vi "Main.vi"() -> ()   [LabVIEW 2013] (continued)
            n2550 = property on="Material Save" class="Bool"("DisabledEnum"=w4223) -> ()  [unwired: 2 in, 2 out]
            n2551 = property class="Clust (strict)"(reference=w4231, "Value"=w4228) -> (reference out=w4227:refnum<vi>)  [unwired: 1 in, 1 out]
            n2552 = local read "DB - Master Data Load"() -> (w4236:bool)
            n2553 = case shown="True" w4236 {
              tunnel: w4227 -> [_ w4239]
              tunnel: w4225 -> [_ w4241]
              frame False {
              }
              frame True {
                w4240 = FALSE  # Include Inactive
                # "Updates Picture"
                # "We will update the [ShortDescription] later during Revision Toggle.\nActually no problem updating here also, but easier to debug code if we\nupdate only in one location."
                # "Updates Rev ComboBox"
                # "Use DB"
                n2554 = local read "Logon"() -> (w4244:T21)
                n2555 = Unbundle By Name(w4244) -> ("LanguageID"=w4243:string)
                n2556 = call "DB - [MasterData].[Material].vi"("DB - Master Data Material Enum"=DB_-_Master_Data_Material_Enum."SELECT [ShortDescription]", "Include Inactive"=w4240, "SRTRS.MasterData.SAPMaterial/Material"="SRTRS.MasterData.SAPMaterial", "[LanguageId]"=w4243, "Update [ShortDescription] to Cluster"=FALSE, "Clust Refnum"=w4239) -> ("SUMMARY"=w4238:errorcluster)  [unwired: 5 in, 4 out]
                n2557 = local write "DB"(w4238) -> ()
                n2558 = disable-structure shown="Disabled" {
                  disable-tunnel: w4241 -> [w4251 _]
                  disable-tunnel: w4238 -> [w4248 _]
                  frame Disabled {
                    n2559 = control-ref of="Master Data Rev"() -> (w4250:refnum<vi>)
                    n2560 = property class="CmbBox"(reference=w4250, error in=w4248, "Value"="") -> (error out=w4247:errorcluster)  [unwired: 1 out]
                    n2561 = property on="Revision Toggle" class="Str"(error in=w4247, "Val(Sgnl)"=w4251) -> (error out=w4249:errorcluster)  [unwired: 1 in, 1 out]
                    n2562 = local write "Property Node Error"(w4249) -> ()
                  }
                  frame Enabled {
                  }
                }
              }
            }
          }
          frame True {
            # "Blank"
          }
        }
      }
      event "Material.Inactive": Value Change {
        n2563 = event-data() -> ("NewVal"=w4252:bool)  [unwired: 1 in, 5 out]
        n2564 = case shown="True" w4252 {
          frame False {
          }
          frame True {
            n2565 = property on="Master Data Material" class="CmbBox"() -> ("Value"=w4257:string)  [unwired: 2 in, 2 out]
            n2566 = property on="Master Data Rev" class="CmbBox"() -> ("Value"=w4256:string)  [unwired: 2 in, 2 out]
            n2567 = call "String - Create comma seperated String.vi"("B"=w4256, "A"=w4257) -> ("A, B , C (auto comma)"=w4255:string)  [unwired: 9 in]
            n2568 = call "Msgbox - Message Handler.vi"("Short Description (When DB Not Available)"="Inactive Material", "Description (When DB Not Available)"=" cannot be used after inactive. Do you wish to proceed?", "Pre-Description"=w4255, "<.?....> Message Code"="<W 504>") -> ("MHandler Error"=w4253:errorcluster, "OK Out"=w4254:bool)  [unwired: 5 in, 1 out]
            n2569 = local write "MHandler"(w4253) -> ()
            n2570 = property on="Inactive" class="Bool (strict)"("Value"=w4254) -> ()  [unwired: 2 in, 2 out]
          }
        }
      }
      event "Revision Toggle": Value Change {
        # "Called by who?\nIf called by Rev"
        # "Called by either \nItem Details.Order No OR\nItem Details.Revision OR\nMaterial.Master Data Rev"
        n2571 = event-data() -> ("NewVal"=w4261:string)  [unwired: 1 in, 5 out]
        n2572 = case shown="\"Master Data Material\", \"Master Data Rev\"" w4261 {
          tunnel: [w4332 w4345] -> w4271
          tunnel: [w4339 w4344] -> w4269
          tunnel: [w4338 w4343] -> w4270
          tunnel: [w4330 w4342] -> w4267
          tunnel: [w4329 w4341] -> w4266
          tunnel: [w4328 w4340] -> w4262
          frame "Material", "Order No", "Revision", Default {
            w4329 = FALSE  # Include Inactive
            # "Use Buffer because Revsion in Part Details's Item Details  is \n different from Cluster of Rev in Material"
            # "Order No & Parts Details.Revision\nFrom Parts Detail"
            n2573 = control-ref of="Material"() -> (w4333:refnum<vi>)
            n2574 = control-ref of="Setup Thermocouple Location"() -> (w4338:refnum<vi>)
            n2575 = control-ref of="Material Description"() -> (w4339:refnum<vi>)
            n2576 = control-ref of="Material Buffer"() -> (w4334:refnum<vi>)
            n2577 = property on="Revision" class="CmbBox"() -> ("Value"=w4328:string)  [unwired: 2 in, 2 out]
            n2578 = property class="Clust (strict)"(reference=w4334) -> (reference out=w4337:refnum<vi>, "Value"=w4335:T12)  [unwired: 1 in, 1 out]
            n2579 = property on="Material" class="CmbBox"(reference=w4333) -> (reference out=w4332:refnum<vi>, "Value"=w4331:string)  [unwired: 1 in, 1 out]
            n2580 = Bundle By Name(cluster=w4335, "Master Data Material"=w4331, "Master Data Rev"=w4328) -> (w4336:T12)
            n2581 = property class="Clust (strict)"(reference=w4337, "Value"=w4336) -> (reference out=w4330:refnum<vi>)  [unwired: 1 in, 1 out]
          }
          frame "Master Data Material", "Master Data Rev" {
            w4341 = TRUE  # Include Inactive
            # "From Material.Master Data Rev"
            n2582 = control-ref of="Master Data Material Description"() -> (w4344:refnum<vi>)
            n2583 = control-ref of="Master Data Thermocouple Location"() -> (w4343:refnum<vi>)
            n2584 = control-ref of="Master Data Material"() -> (w4345:refnum<vi>)
            n2585 = control-ref of="Material"() -> (w4342:refnum<vi>)
            n2586 = property on="Master Data Rev" class="CmbBox"() -> ("Value"=w4340:string)  [unwired: 2 in, 2 out]
          }
        }
        n2587 = local read "DB - Master Data Load"() -> (w4268:bool)
        n2588 = property on="Material" class="CmbBox"(reference=w4271) -> ("Value"=w4272:string)  [unwired: 1 in, 2 out]
        n2589 = case shown="True" w4268 {
          tunnel: [w4279 w4314] -> w4273
          tunnel: w4272 -> [w4281 _]
          tunnel: w4269 -> [w4280 w4301]
          tunnel: w4267 -> [_ w4313]
          tunnel: w4266 -> [_ w4312]
          tunnel: [w4277 w4311] -> w4265
          tunnel: [w4275 w4310] -> w4264
          tunnel: w4262 -> [w4274 _]
          frame False {
            w4293 = "_" ("string")
            n2590 = Concatenate Strings(w4281, w4293, w4274, w4293) -> (w4286:string)
            n2591 = local read "MasterData\\JPG"() -> (w4290:path)
            n2592 = Concatenate Strings(w4286, "*.jpg" ("string")) -> (w4285:string)
            n2593 = List Folder(path=w4290, pattern=w4285) -> (filenames=w4292:string[])  [unwired: 2 in, 3 out]
            n2594 = Index Array(array=w4292, index=0) -> (element=w4288:string)
            n2595 = Build Path(base path=w4290, name or relative path=w4288) -> (appended path=w4289:path)
            n2596 = Match Pattern(string=w4288, regular expression=w4286) -> (after substring=w4284:string)  [unwired: 1 in, 3 out]
            n2597 = Match Pattern(string=w4284, regular expression="[.]") -> (before substring=w4282:string)  [unwired: 1 in, 3 out]
            n2598 = property class="Str"(reference=w4280, "Value"=w4282) -> (reference out=w4278:refnum<vi>)  [unwired: 1 in, 1 out]
            n2599 = call <vilib>:"Check if File or Folder Exists.vi"("path"=w4289) -> ("file or folder exists?"=w4279:bool, "dup path"=w4276:path)  [unwired: 8 in, 1 out]
            n2600 = case shown="True" w4279 {
              tunnel: w4278 -> [w4294 _]
              tunnel: w4276 -> [_ w4297]
              tunnel: [_ w4296] -> w4277
              frame False {
                # "File Does Not Exist"
                n2601 = invoke class="Str" method="Reinit To Default"(reference=w4294) -> ()  [unwired: 2 in, 3 out]
              }
              frame True {
                n2602 = local write "MasterData Image File Path"(w4297) -> ()
                n2603 = call <vilib>:"Read JPEG File.vi"("path to JPEG file"=w4297) -> ("error out"=→"Material Image File":errorcluster, "image data"=w4296:T40)  [unwired: 8 in, 1 out]
              }
            }
            n2604 = Path To String(path=w4276) -> (string=w4275:string)
          }
          frame True {
            # "Update Description only if Rev is Blank"
            # "Use DB"
            n2605 = local read "Logon"() -> (w4308:T21)
            n2606 = Unbundle By Name(w4308) -> ("LanguageID"=w4307:string)
            n2607 = call "DB - [MasterData].[Material].vi"("DB - Master Data Material Enum"=DB_-_Master_Data_Material_Enum."SELECT [Description], [ImageFile]", "Include Inactive"=w4312, "[LanguageId]"=w4307, "Clust Refnum"=w4313) -> ("image data"=w4311:T40, "ImageFile OK"=w4314:bool, "Material File"=w4309:path, "SUMMARY"=w4316:errorcluster)  [unwired: 7 in, 1 out]
            n2608 = property class="Clust (strict)"(reference=w4313, error in=w4316) -> (error out=w4304:errorcluster, "Value"=w4315:T12)  [unwired: 1 out]
            n2609 = Unbundle By Name(w4315) -> ("Master Data Material Description"=w4302:string)
            n2610 = disable-structure shown="Enabled" {
              disable-tunnel: w4302 -> [w4325 _]
              disable-tunnel: [w4324 T30."Enabled" ("Disabled")] -> w4299
              disable-tunnel: [w4318 u32 16777215] -> w4298
              frame Disabled {
                n2611 = Empty String/Path?(string/path=w4325) -> (empty?=w4321:bool)
                n2612 = Select(t=u32 16777215, s=w4321, f=u32 16250871) -> (s? t:f=w4318:u32)
                n2613 = Select(t=T30."Enabled" ("Disabled"), s=w4321, f=T30."Disabled" ("Disabled")) -> (s? t:f=w4324:T30)
              }
              frame Enabled {
              }
            }
            n2614 = local write "MasterData Image File Path"(w4309) -> ()
            n2615 = local read "Logon Extra"() -> (w4306:T25)
            n2616 = property class="Str"(reference=w4301, "DisabledEnum"=w4299, "Text.BGColor"=w4298) -> (reference out=w4300:refnum<vi>)  [unwired: 1 in, 1 out]
            n2617 = Unbundle By Name(w4306) -> ("IsUnicode"=w4305:bool)
            n2618 = call "Tool_Unicode Update String.vi"("Interpret as Unicode (T)"=w4305, "error in (no error)"=w4304, "String Value"=w4302, "String Control Reference"=w4300) -> ("error out"=w4303:errorcluster)  [unwired: 4 in, 1 out]
            n2619 = local write "Material Image File"(w4303) -> ()
            n2620 = Path To String(path=w4309) -> (string=w4310:string)
          }
        }
        n2621 = case shown="True" w4273 {
          tunnel: w4270 -> [w4348 w4355]
          tunnel: w4265 -> [_ w4352]
          tunnel: w4264 -> [_ w4351]
          tunnel: [w4346 w4350] -> w4263
          frame False {
            # "No Image"
            n2622 = disable-structure shown="Disabled" {
              frame Disabled {
                n2623 = property on="Material Save" class="Bool"("DisabledEnum"=T30."Disabled and Grayed Out" ("Disabled")) -> ()  [unwired: 2 in, 2 out]
              }
              frame Enabled {
              }
            }
            n2624 = invoke class="Pict" method="Reinit To Default"(reference=w4348) -> (error out=w4346:errorcluster)  [unwired: 2 in, 2 out]
            n2625 = property on="Material Copy" class="Bool"("DisabledEnum"=T30."Disabled and Grayed Out" ("Disabled")) -> ()  [unwired: 2 in, 2 out]
          }
          frame True {
            # "Valid Image File"
            n2626 = disable-structure shown="Disabled" {
              frame Disabled {
                n2627 = property on="Material Save" class="Bool"("DisabledEnum"=T30."Enabled" ("Disabled")) -> ()  [unwired: 2 in, 2 out]
              }
              frame Enabled {
              }
            }
            n2628 = call <vilib>:"Draw Flattened Pixmap.vi"("image data"=w4352, "picture"=picture data[5B]) -> ("new picture"=w4356:picture)  [unwired: 7 in]
            n2629 = property on="Material Copy" class="Bool"("DisabledEnum"=T30."Enabled" ("Disabled")) -> ()  [unwired: 2 in, 2 out]
            n2630 = property on="Property Node" class="Pict"(reference=w4355, "Value"=w4356, "Desc"=w4351) -> (error out=w4350:errorcluster)  [unwired: 1 in, 1 out]
          }
        }
        n2631 = local write "Material Image File"(w4263) -> ()
      }
    }
    "UI Event" <- w479
  }
  n2632 = while {
    shift-right: [w4366] -> _
    shift-left: w25 -> [w4363]
    shift-right: [w4367] -> w7
    shift-left: w24 -> [w4372]
    shift-right: [w4368] -> _
    shift-left: w15 -> [w4369]
    tunnel: w20 -> [_]
    shift-left: w1 -> [w4364]
    shift-right: [w4361] -> _
    shift-left: w13 -> [w4362]
    shift-right: [w4360] -> _
    shift-left: w12 -> [w4359]
    stop <- w4365 stop-if-true
    # "StateMachine For MainProcess                                                         StateMachine For MainProcess                                                         StateMachine For MainProcess                                                         StateMachine For MainProcess                                                         StateMachine For MainProcess                                                         StateMachine For MainProcess                                                         StateMachine For MainProcess"
    n2633 = case shown="\"END Recipe\"" w4363 {
      selector: w4363 -> [w4391 _ _ _ w5684 _ _ _ _ w6675]
      tunnel: [w4382 w5238 Enum_-_SRTRS_State."BEGIN Process" ("Enum") Enum_-_SRTRS_State."RUNNING Process" ("Enum") w5685 Enum_-_SRTRS_State."Spare Enum" ("Enum") Enum_-_SRTRS_State."END Recipe" ("Enum") Enum_-_SRTRS_State."READY TO START" ("Enum") w6608 w6675] -> w4371
      tunnel: [w4388 w5228 _ w5569 w5670 w6212 _ w6264 _ _] -> w4367
      tunnel: w4372 -> [_ _ _ _ _ w6212 _ _ w6606 _]
      tunnel: [_ _ _ _ _ _ _ _ w6607 TRUE] -> w4365
      tunnel: w4369 -> [w4385 _ _ _ w5661 _ _ _ w6604 _]
      tunnel: [w4389 0 _ w5565 w5678 _ 0 _ w6604 _] -> w4368
      tunnel: w4364 -> [w4390 _ _ _ _ _ _ _ w6605 _]
      tunnel: w4362 -> [_ _ _ _ w5676 _ _ _ w6603 _]
      tunnel: [_ _ _ ET3500_Program_Status."Wait For RUN" w5675 _ _ _ w6603 _] -> w4361
      tunnel: [_ _ _ _ w5673 _ _ _ w6602 _] -> w4360
      tunnel: w4359 -> [_ _ _ _ w5672 _ _ _ w6602 _]
      frame "READY TO START", Default {
        (unwired) FALSE  # RecoveryFlag only checked at "Execute" Page
        # "This wil be checked again at \"Start Cycle\" to prevent resending of DAQ Start"
        # "Setup, Default\nLogon\nExecute"
        n2634 = flat-sequence {
          frame #0 {
            # "Check if Transaction Number is Empty"
            n2635 = local read "Transaction No"() -> (w4397:string)
            n2636 = Empty String/Path?(string/path=w4397) -> (empty?=w4396:bool)
            n2637 = Select(t=T30."Disabled and Grayed Out" ("Disabled"), s=w4396, f=T30."Enabled" ("Disabled")) -> (s? t:f=w4398:T30)
            n2638 = property on="Recipe Start" class="Bool"("DisabledEnum"=w4398) -> ()  [unwired: 2 in, 2 out]
            n2639 = property on="Close" class="Bool (strict)"("DisabledEnum"=T30."Enabled" ("Disabled")) -> ()  [unwired: 2 in, 2 out]
          }
        }
        n2640 = local read "Tab Body"() -> (w4387:T1)
        n2641 = Equal?(x=w4391, y=w4390) -> (x = y?=w4386:bool)
        n2642 = case shown="\"Logon\"" w4387 {
          selector: w4387 -> [_ w4981]
          tunnel: [w4406 w4986] -> w4389
          tunnel: [w4405 w4985] -> w4383
          tunnel: [_ w4984] -> w4388
          tunnel: w4386 -> [_ _]
          tunnel: w4385 -> [_ _]
          frame "Logon" {
            w4405 = FALSE  # RecoveryFlag only checked at "Setup" Tab
            w4406 = 0  # Resets Sample/ch count
            # "\"ini\" Settings to be loaded here"
            n2643 = local read "Logon OK"() -> (w4404:bool)
            n2644 = case shown="True" w4404 {
              frame False {
                # "Check Logon OK"
                n2645 = flat-sequence {
                  tunnel: [w4413] -> w4409
                  tunnel: w4409 -> [w4420]
                  tunnel: [w4421] -> w4408
                  tunnel: [w4420] -> w4407
                  tunnel: w4408 -> [w4422]
                  tunnel: w4407 -> [w4423]
                  frame #0 {
                    n2646 = control-ref of="Logon OK"() -> (w4411:refnum<vi>)
                    n2647 = control-ref of="[RawDataReport]"() -> (w4410:refnum<vi>)
                    n2648 = control-ref of="Logon"() -> (w4412:refnum<vi>)
                    n2649 = control-ref of="Logon Extra"() -> (w4416:refnum<vi>)
                    n2650 = control-ref of="[TabUserAccess]"() -> (w4414:refnum<vi>)
                    n2651 = local read "Logon UI"() -> (w4413:refnum<vi>)
                    n2652 = Build Array(w4411, w4412, w4416, w4414, w4410) -> (w4415:refnum<vi>[])
                    n2653 = for {
                      tunnel: w4413 -> [w4419]
                      tunnel: w4415 -> [w4418] mode=indexing
                      n2654 = call "subPanel - Read Value.vi"("subPanel Ref"=w4419, "CtlRef"=w4418) -> ("Error Out"=w4417:errorcluster)  [unwired: 6 in, 3 out]
                      n2655 = local write "SubPanel"(w4417) -> ()
                    }
                  }
                  frame #1 {
                    # "SET GLOBAL SRTRS to Logon Parameters"
                    n2656 = local read "Logon OK"() -> (w4421:bool)
                  }
                  frame #2 {
                    n2657 = case shown="True" w4422 {
                      tunnel: w4423 -> [_ w4431]
                      frame False {
                      }
                      frame True {
                        # "Logon UI should already be closed"
                        n2658 = control-ref of="Logon UI"() -> (w4432:refnum<vi>)
                        n2659 = Close Reference(reference=w4431) -> (error out=w4433:errorcluster)  [unwired: 1 in]
                        n2660 = invoke on="Invoke Node" class="SubPnl" method="Remove VI"(reference=w4432, error in=w4433) -> (error out=→"SubPanel":errorcluster)  [unwired: 1 in, 2 out]
                        n2661 = global write "Global SRTRS.vi" "[RawDataReport]"("[RawDataReport]") -> ()
                        n2662 = global write "Global SRTRS.vi" "Logon Extra"("Logon Extra") -> ()
                        n2663 = global write "Global SRTRS.vi" "Logon"("Logon") -> ()
                        n2664 = Unbundle By Name("Logon") -> ("PlantID"=w4428:string, "UserID"=w4426:string)
                        n2665 = disable-structure shown="Enabled" {
                          disable-tunnel: w4426 -> [w4436 _]
                          disable-tunnel: "Logon Extra" -> [_ _]
                          disable-tunnel: "Logon" -> [_ _]
                          frame Enabled {
                            n2666 = call "Msgbox - Message Handler.vi"("Short Description (When DB Not Available)"="Logon Successful", "Description (When DB Not Available)"=" logon successful." ("Short Description (When DB Not Available)"), "Pre-Description"=w4436, "<.?....> Message Code"="<I 101>") -> ("MHandler Error"=w4437:errorcluster)  [unwired: 5 in, 2 out]
                            n2667 = local write "MHandler"(w4437) -> ()
                          }
                          frame Disabled {
                          }
                        }
                        n2668 = local write "User"(w4426) -> ()
                        n2669 = String Length(string=w4428) -> (length=w4427:i32)
                        n2670 = case shown="0" w4427 {
                          tunnel: "Logon Extra" -> [_ _]
                          frame 0 {
                            w4439 = FALSE
                            # "No PlantId\nDB Failed. Disable all DB."
                            n2671 = local write "DB - Master Data Save"(w4439) -> ()
                            n2672 = local write "DB - Master Data Load"(w4439) -> ()
                            n2673 = local write "DB - Setup Item (Part Details)"(w4439) -> ()
                            n2674 = local write "DB - Transaction"(w4439) -> ()
                            n2675 = local write "DB - Logon"(w4439) -> ()
                            n2676 = local write "DB - Report"(w4439) -> ()
                            n2677 = local write "DB - Message"(w4439) -> ()
                            n2678 = local write "DB - Active Process"(w4439) -> ()
                            n2679 = global write "Global SRTRS.vi" "DB Available"(w4439) -> ()
                            n2680 = call "Msgbox - Message Handler.vi"("Short Description (When DB Not Available)"="Database Not Available", "Description (When DB Not Available)"="Switching to standalone mode" ("Short Description (When DB Not Available)"), "<.?....> Message Code"="<E 107>") -> ("MHandler Error"=w4444:errorcluster, "OK Out"=w4442:bool)  [unwired: 6 in, 1 out]
                            n2681 = local write "MHandler"(w4444) -> ()
                            n2682 = case shown="True" w4442 {
                              frame False {
                                # "Cancel"
                                n2683 = local write "Tab Body"(Enum_-_Tabs."Logon" ("Tab Body")) -> ()
                                n2684 = local write "Logon OK"(FALSE ("Logon OK")) -> ()
                                n2685 = property on="Close" class="Bool (strict)"("BoolText.Text"="Close Now" ("Label.Text")) -> (error out=w4446:errorcluster)  [unwired: 2 in, 1 out]
                                n2686 = property on="Close" class="Bool (strict)"(error in=w4446, "Val(Sgnl)"=TRUE ("Value (Signaling)")) -> ()  [unwired: 1 in, 2 out]
                              }
                              frame True {
                                # "Setup the Folders (Phase1)"
                                # "Hide Logon"
                                # "Proceed with SRTRS with no DB"
                                n2687 = flat-sequence "Edit WPS in Setup" {
                                frame #0 {
                                w4463 = TRUE
                                # "No DB so must let user Edit WPS"
                                n2688 = control-ref of="MCListBox FHS Master Data"() -> (w4470:refnum<vi>)
                                n2689 = control-ref of="MCListBox FHS Setup"() -> (w4469:refnum<vi>)
                                n2690 = case shown="True" w4463 {
                                tunnel: w4470 -> [w4473 w4475]
                                tunnel: [w4474 w4477] -> w4468
                                tunnel: w4469 -> [_ w4476]
                                frame False {
                                # "Only Master FHS"
                                n2691 = Build Array(w4473) -> (w4474:refnum<vi>[])
                                }
                                frame True {
                                # "Both FHS"
                                n2692 = Build Array(w4476, w4475) -> (w4477:refnum<vi>[])
                                }
                                }
                                n2693 = control-ref of="MCListBox FHS Setup Remove Button"() -> (w4467:refnum<vi>)
                                n2694 = control-ref of="MCListBox FHS Setup Add Button"() -> (w4466:refnum<vi>)
                                n2695 = local write "Edit WPS in Setup"(w4463) -> ()
                                n2696 = control-ref of="Tab Setup"() -> (w4464:refnum<vi>)
                                n2697 = local read "CellBG New Cells"() -> (w4471:u32)
                                n2698 = for {
                                tunnel: w4471 -> [w4482]
                                tunnel: w4468 -> [w4479] mode=indexing
                                # "MClistbox FHS Setup \nis set to FALSE for\n\"Allowing Editing Cells\"\n/\"Editable Cells"
                                # "Create WHITE\neditable cells"
                                n2699 = property on="Property Node" class="MCListbox (strict)"(reference=w4479, "Allow Editing Cells"=TRUE) -> (reference out=w4481:refnum<vi>, "NumCols"=w4480:u32)  [unwired: 1 in, 1 out]
                                n2700 = for {
                                N: w4480 -> [_]
                                tunnel: w4482 -> [w4484]
                                tunnel: w4481 -> [w4483]
                                i -> [w4486]
                                n2701 = Bundle("Multicolumn Listbox"=0, w4486) -> (w4485:cluster{"Multicolumn Listbox":i32, i32})  [unwired: 1 in]
                                n2702 = property on="Property Node" class="MCListbox (strict)"(reference=w4483, "ActiveCell"=w4485, "CellBG"=w4484) -> ()  [unwired: 1 in, 2 out]
                                }
                                }
                                n2703 = control-ref of="No."() -> (w4472:refnum<vi>)
                                n2704 = property class="Bool"(reference=w4467, "Visible"=w4463) -> ()  [unwired: 1 in, 2 out]
                                n2705 = property class="Bool"(reference=w4466, "Visible"=w4463) -> ()  [unwired: 1 in, 2 out]
                                n2706 = call "Setup Tab - Enable-Disable.vi"("No."=w4472, "[SRTRS][Config][ParameterSettings] - [userEditableProcedure]"=w4463, "Disabled"=T30."Enabled", "Tab Setup"=w4464) -> ()  [unwired: 8 in]
                                }
                                }
                                n2707 = local read "SRTRS4070 Folder (Server Folder)"() -> (w4451:string)
                                n2708 = local read "SRTRS4070 Host Folder"() -> (w4450:string)
                                n2709 = property on="Mytab" class="TabCtl (strict)"() -> ("Pages"=w4455:refnum<vi>[])  [unwired: 2 in, 2 out]
                                n2710 = call "Folder - Get Application Folders Ref.vi"("Pages"=w4455) -> ("Host Paths"=w4457:refnum<vi>[], "Paths"=w4456:refnum<vi>[])  [unwired: 9 in]
                                n2711 = control-ref of="Tab Body"() -> (w4459:refnum<vi>)
                                n2712 = call "Folder - Create Application Folders.vi"("ControlsOnPage"=w4456, "SRTRS4070 Folder"=w4451) -> ("error out"=w4453:errorcluster)  [unwired: 8 in, 1 out]
                                n2713 = call "Folder - Create Application Folders.vi"("ControlsOnPage"=w4457, "SRTRS4070 Folder"=w4450) -> ()  [unwired: 8 in, 2 out]
                                n2714 = call "Tabs - Page Visibility.vi"("Matching Tab#"=i32[] [0, 1, 2, 3, 11, 12, 20], "PageLabel"=string[] ["Setup", "Execute", "Report", "Master Data", "Admin", "Config", "Logon"], "[TabUserAccess]"=bool[] [TRUE, TRUE, TRUE, TRUE, FALSE, FALSE, FALSE], "TabControl in"=w4459) -> ("Error Out"=w4458:errorcluster)  [unwired: 7 in]
                                n2715 = property on="Data" class="Path"(error in=w4453) -> (error out=w4454:errorcluster, "Value"=w4452:path)  [unwired: 1 in, 1 out]
                                n2716 = flat-sequence {
                                tunnel: w4458 -> [_]
                                frame #0 {
                                # "Must Make Tabs Visible B4 we Set the Tab to show"
                                n2717 = local write "Tab Body"(Enum_-_Tabs."Setup" ("Tab Body")) -> ()
                                }
                                }
                                n2718 = property on="Raw Data File (Report Tab)" class="Path"(error in=w4454, "StartPath"=w4452) -> ()  [unwired: 1 in, 2 out]
                              }
                            }
                          }
                          frame 1, Default {
                          }
                        }
                      }
                    }
                  }
                }
              }
              frame True {
                # "Proceed with Normal Start at Setup TAB\nChange Close Boolean Text to \"Log off\""
                n2719 = local read "Settings Load Sequence"() -> (w4489:i32[])
                n2720 = for {
                  tunnel: w4489 -> [w4490] mode=indexing
                  n2721 = case shown="..0" w4490 {
                    frame ..0 {
                      w4527 = ""
                      w4535 = 1  # [Description]
                      w4537 = 6  # [SoftwareSolutionId]
                      w4543 = 0  # [OutputSetId]
                      w4542 = 0  # 1st row (sorted in SQL)
                      w4566 = 1  # [ChannelMapping]
                      w4567 = 0  # [IpAddress]
                      w4578 = "01"  # [UnitOfMeasurementId]
                      w4587 = 4  # [ClientFilePath]
                      w4588 = 3  # [FileServerPath]
                      w4590 = 1  # [TimeZone]
                      w4591 = 2  # [Software Solution Name]
                      w4609 = 0  # [LogoFile]
                      w4526 = ", " ("string")
                      # "2015-01-01 11:19\n[Furnace Serial No]                        [Eurotherm]                 [Model]                                     [Description]                            [Equipment Serial No]                  [EquipmentId]                [LastCalibDate]                         [NextCalibDate]                   8  [NoticePeriod]                          [IsCalibRequired]"
                      # "Used by DB - Config Messages"
                      # "SQL Script:\nFORMAT(b.[LastCalibDate], 'yyyy-MM-dd')\nFORMAT(b.[NextCalibDate], 'yyyy-MM-dd')"
                      # "We need the Date Format for \n- Furnace Details and\n- Equipment Details\nSo we get it here 1st. The rest of the Config Parameters will be grabbed in Sequence 1.\nDate Format will be read again in Sequence 1, for easy code maintanence."
                      # "Plant Name, SystemId, UserName"
                      # "No , if Blank"
                      # "Legacy: No OPEN and CLOSE in Col Info"
                      # "Updates Local/Global Variables"
                      n2722 = global read "Global SRTRS.vi" "Logon Extra"() -> (w4524:T25)
                      n2723 = global read "Global SRTRS.vi" "Logon"() -> (w4546:T21)
                      n2724 = global read "Global SRTRS.vi" "SRTRS Connection Information"() -> (w4604:T38)
                      n2725 = disable-structure shown="Disabled" {
                        frame Disabled {
                          n2726 = control-ref of="Material"() -> ()  [unwired: 1 out]
                          n2727 = control-ref of="Revision"() -> ()  [unwired: 1 out]
                          n2728 = control-ref of="Qty."() -> ()  [unwired: 1 out]
                          n2729 = control-ref of="Oper. No."() -> ()  [unwired: 1 out]
                          n2730 = control-ref of="NCR No."() -> ()  [unwired: 1 out]
                          n2731 = control-ref of="Customer No."() -> ()  [unwired: 1 out]
                          n2732 = control-ref of="Customer Name"() -> ()  [unwired: 1 out]
                          n2733 = control-ref of="Project"() -> ()  [unwired: 1 out]
                          n2734 = control-ref of="Sales Order"() -> ()  [unwired: 1 out]
                          n2735 = control-ref of="Item No."() -> ()  [unwired: 1 out]
                          n2736 = control-ref of="Material Description"() -> ()  [unwired: 1 out]
                          n2737 = control-ref of="Serial No."() -> ()  [unwired: 1 out]
                          n2738 = control-ref of="UnitOfQty"() -> ()  [unwired: 1 out]
                        }
                        frame Enabled {
                        }
                      }
                      n2739 = Unbundle By Name(w4524) -> ("Hostname [ClientName]"=w4539:string)
                      n2740 = Unbundle By Name(w4524) -> ("IsUnicode"=w4498:bool)
                      n2741 = control-ref of="Material Description"() -> (w4521:refnum<vi>)
                      n2742 = control-ref of="Customer Name"() -> (w4523:refnum<vi>)
                      n2743 = control-ref of="Project"() -> (w4522:refnum<vi>)
                      n2744 = control-ref of="Notes"() -> (w4520:refnum<vi>)
                      n2745 = Unbundle By Name(w4546) -> ("PlantID"=w4548:string, "StationID"=w4547:string)
                      n2746 = call "DB - [Setup].[Item] (Part Details).vi"("DB - Setup Item Enum"=DB_-_Setup_Item_Enum."SELECT [Plant],[OrderNo]", "DB.Schema.Table Array"=string[] ["SRTRS.Config.Mapping"], "OrderNo"="") -> ("[IsMandatory] Ordered"=→"[IsMandatory]":string[])  [unwired: 7 in, 5 out]
                      n2747 = call "DB - [Config].[StationSysRelation].vi"("[ClientName]"=w4539, "[StationId]"=w4547, "[PlantId]"=w4548) -> ("[SystemId]"=w4533:string)  [unwired: 6 in, 2 out]
                      n2748 = Build Array(w4523, w4522, w4521, w4520) -> (w4519:refnum<vi>[])
                      n2749 = Bundle By Name(cluster=w4546, "SystemID"=w4533) -> (w4510:T21)
                      n2750 = Unbundle By Name(w4510) -> ("PlantID"=w4501:string, "LanguageID"=w4499:string)
                      n2751 = Unbundle By Name(w4604) -> ("Connection"=w4603:string, "Username"=w4602:string, "Password"=w4601:string)
                      n2752 = call "DB - [Config].[SoftwareSolution].vi"("[LanguageId]"=w4499, "Application"="SRTRS", "[PlantId]"=w4501) -> ("1D data"=w4610:string[])  [unwired: 6 in, 2 out]
                      n2753 = property on="SystemID" class="Str"("Value"=w4533) -> ()  [unwired: 2 in, 2 out]
                      n2754 = Unbundle By Name(w4510) -> ("PlantID"=w4516:string)
                      n2755 = Format Into String(DB_-_[Config].[Parameters].[ParameterId]_Values."DateFormat" ("v20140926_1200")) -> (resulting string=w4506:string)  [unwired: 3 in, 1 out]
                      n2756 = for {
                        tunnel: w4498 -> [w4633]
                        tunnel: w4519 -> [w4632] mode=indexing
                        n2757 = call "Tool_Unicode Property Interpret As Unicode.vi"("Interpret As Unicode (T)"=w4633, "String Control Reference"=w4632) -> ()  [unwired: 6 in, 2 out]
                      }
                      n2758 = Unbundle By Name(w4510) -> ("LanguageID"=w4589:string, "PlantID"=w4570:string, "SystemID"=w4569:string)
                      n2759 = Build Array(w4506) -> (w4505:string[])
                      n2760 = Index Array(array=w4610, index #1=w4609, index #2=w4590, index #3=w4591, index #4=w4588, index #5=w4587, index #6=w4537) -> (element #1=w4538:string, element #2=→"[TimeZone]":string, element #3=w4495:string, element #4=w4586:string, element #5=w4583:string, element #6=w4536:string)
                      "[LogoFile]" <- w4538
                      n2761 = call-poly <vilib>:"DB Tools Open Connection.vi"("password"=w4601, "userID"=w4602, "connection information"=w4603) -> ("error out"=w4599:errorcluster, "connection reference"=w4600:T66)  [unwired: 5 in]
                      n2762 = global write "Global SRTRS.vi" "Logon"(w4510) -> ()
                      n2763 = call "DB - [Config].[Parameter].vi"("Application"="SRTRS", "[PlantId]"=w4501, "[ParameterId] Values"=w4505) -> ("2D data"=w4503:string[][])  [unwired: 6 in, 2 out]
                      n2764 = global write "Global SRTRS.vi" "[SoftwareSolutionId]"(w4536) -> ()
                      n2765 = String To Path(string=w4538) -> (path=w4606:path)
                      n2766 = call "DB - Columns INFO.vi"("Refnum in"=w4600, "DB.dbo.Table"="SRTRS.Setup.Item", "error in (no error)"=w4599) -> ("Refnum out"=w4597:T66, "COLUMN_NAME"=→"[Setup].[Item] COLUMN_NAME":string[], "DATA_TYPE"=→"[Setup].[Item] DATA_TYPE":string[], "PRECISION"=→"[Setup].[Item] PRECISION":string[], "error out"=w4598:errorcluster)  [unwired: 4 in, 4 out]
                      n2767 = global read "Global SRTRS.vi" "Logon Extra"() -> (w4572:T25)
                      n2768 = local write "SRTRS4070 Host Folder"(w4583) -> ()
                      n2769 = local write "SRTRS4070 Folder (Server Folder)"(w4586) -> ()
                      n2770 = call <vilib>:"Read JPEG File.vi"("path to JPEG file"=w4606) -> ("error out"=w4605:errorcluster, "image data"=w4608:T40)  [unwired: 8 in, 1 out]
                      n2771 = Index Array(array=w4503, index (row)=0 ("disabled index (col)"), index (col)=1 ("disabled index (col)")) -> (element=w4494:string)
                      n2772 = call "DB - [Config].[Controller].vi"("[SystemId]"=w4569, "[PlantId]"=w4570) -> ("data"=w4568:string[])  [unwired: 7 in, 2 out]
                      n2773 = local write "LogoName"(w4605) -> ()
                      n2774 = call <vilib>:"DB Tools Close Connection.vi"("error in (no error)"=w4598, "connection reference"=w4597) -> ("error out"=w4592:errorcluster)  [unwired: 5 in]
                      n2775 = call <vilib>:"Draw Flattened Pixmap.vi"("image data"=w4608) -> ("new picture"=w4607:picture)  [unwired: 8 in]
                      n2776 = property on="Mytab" class="TabCtl (strict)"() -> ("Pages"=w4585:refnum<vi>[])  [unwired: 2 in, 2 out]
                      n2777 = local write "Date Format (UserDefined)"(w4494) -> ()
                      n2778 = global write "Global SRTRS.vi" "[SoftwareSolutionName]"(w4495) -> ()
                      n2779 = local write "LogoName"(w4607) -> ()
                      n2780 = Unbundle By Name(w4572) -> ("Plant Name"=w4532:string, "UserName"=w4616:string)
                      n2781 = call "Folder - Get Application Folders Ref.vi"("Pages"=w4585) -> ("Host Paths"=w4582:refnum<vi>[], "Paths"=w4584:refnum<vi>[])  [unwired: 9 in]
                      n2782 = Unbundle By Name(w4510) -> ("SystemID"=w4529:string, "UserID"=w4619:string)
                      n2783 = Index Array(array=w4568, index #1=w4567, index #2=w4566) -> (element #1=w4556:string, element #2=w4562:string)
                      n2784 = local write "DB"(w4592) -> ()
                      n2785 = call "DB - [MasterData].[OutputSet].vi"("Master Data OuputSet SQL"=DB_-_Master_Data_OutputSet_SQL."SELECT [OutputSetId]", "DB Connection"=T53 {"Open"=TRUE, "Close"=TRUE}, "[PlantId]"=w4516) -> ("SUMMARY"=w4517:errorcluster, "2D data"=w4544:string[][], "connection reference"=w4514:T66)  [unwired: 4 in, 2 out]
                      n2786 = call "Folder - Create Application Folders.vi"("ControlsOnPage"=w4584, "SRTRS4070 Folder"=w4586) -> ("error out"=w4577:errorcluster)  [unwired: 8 in, 1 out]
                      n2787 = call "Folder - Create Application Folders.vi"("ControlsOnPage"=w4582, "SRTRS4070 Folder"=w4583) -> ("error out"=w4576:errorcluster)  [unwired: 8 in, 1 out]
                      n2788 = Bundle("String"=w4562) -> (w4534:cluster{"String":string})  [unwired: 1 in]
                      n2789 = call "DB - [Config].[System].vi"("[LanguageId]"=w4589, "Date Format (User Defined)"=w4494, "AND IN (EquipmentIDx,..)"=FALSE, "[PlantId]"=w4570, "[SystemId]"=w4569) -> ("Furnace Details"=w4493:T6, "Equipment Details (Itemnames)"=w4492:string[][])  [unwired: 7 in, 2 out]
                      n2790 = local write "User"(w4619) -> ()
                      n2791 = flat-sequence {
                        tunnel: w4577 -> [_]
                        tunnel: w4576 -> [_]
                        frame #0 {
                          n2792 = local read "MasterData\\JPG"() -> (w4644:path)
                          n2793 = local read "MasterData\\Layout"() -> (w4643:path)
                          n2794 = global write "Global SRTRS.vi" "Server MasterData\\JPG Folder"(w4644) -> ()
                          n2795 = global write "Global SRTRS.vi" "Server MasterData\\Layout Folder"(w4643) -> ()
                        }
                      }
                      n2796 = Index Array(array=w4544, index (row) #1=w4542, index (col) #1=w4543, index (row) #2=w4542, index (col) #2=w4535) -> (element #1=w4515:string, element #2=w4541:string)
                      n2797 = local write "Channel to Probe Mapping"(w4534) -> ()
                      n2798 = Empty String/Path?(string/path=w4532) -> (empty?=w4531:bool)
                      n2799 = control-ref of="ApplicationName"() -> (w4497:refnum<vi>)
                      n2800 = property on="Equipment Details" class="MCListbox (strict)"("ItemNames"=w4492) -> ()  [unwired: 2 in, 2 out]
                      n2801 = Bundle("String"=w4515, "String"=w4541) -> (w4540:cluster{"String":string, "String":string})  [unwired: 1 in]
                      n2802 = property on="Furnace Details" class="Clust (strict)"("Value"=w4493) -> ()  [unwired: 2 in, 2 out]
                      n2803 = Empty String/Path?(string/path=w4529) -> (empty?=w4528:bool)
                      n2804 = Unbundle By Name(w4510) -> ("StationID"=w4509:string)
                      n2805 = call "Tool_Unicode Update String.vi"("Interpret as Unicode (T)"=TRUE, "String Value"=w4495, "String Control Reference"=w4497) -> ()  [unwired: 5 in, 2 out]
                      n2806 = property on="Results Output" class="Clust (strict)"("Value"=w4540) -> ()  [unwired: 2 in, 2 out]
                      n2807 = Concatenate Strings("cRIO IP = " ("string"), w4556, " [ChannelMapping] = " ("string"), w4562) -> (w4512:string)
                      n2808 = Select(t=w4527, s=w4531, f=w4526) -> (s? t:f=w4530:string)
                      n2809 = Select(t=w4527, s=w4528, f=w4526) -> (s? t:f=w4525:string)
                      n2810 = Empty String/Path?(string/path=w4509) -> (empty?=w4508:bool)
                      n2811 = disable-structure shown="Disabled" {
                        disable-tunnel: w4517 -> [w4629 _]
                        disable-tunnel: w4516 -> [w4628 _]
                        disable-tunnel: w4515 -> [w4627 _]
                        disable-tunnel: w4514 -> [w4623 _]
                        frame Disabled {
                          # "Write to ini file"
                          n2812 = call "DB - [MasterData].[OutputSet].vi"("Master Data OuputSet SQL"=DB_-_Master_Data_OutputSet_SQL."SELECT [LayoutFilePath],[LayoutFileName]", "DB Connection"=T53 {"Open"=FALSE, "Close"=TRUE}, "error in (no error)"=w4629, "[PlantId]"=w4628, "[OutputSetId]"=w4627, "connection reference"=w4623) -> ("Template Files"=w4625:string[], "[LayoutId]"=w4626:string[])  [unwired: 1 in, 3 out]
                          n2813 = Build Array(w4626, w4625) -> (w4624:string[][])
                          n2814 = Transpose 2D Array(2D array=w4624) -> ()  [unwired: 1 out]
                        }
                        frame Enabled {
                        }
                      }
                      n2815 = property on="Close" class="Bool (strict)"("BoolText.Text"="Log off") -> ()  [unwired: 2 in, 2 out]
                      n2816 = Concatenate Strings(w4532, w4530, w4529, w4525, w4616) -> (w4622:string)
                      n2817 = flat-sequence "Report TAB" {
                        tunnel: w4508 -> [w4635]
                        frame #0 {
                          n2818 = global read "Global SRTRS.vi" "[RawDataReport]"() -> (w4637:bool)
                          n2819 = Select(t=T30."Enabled" ("Disabled"), s=w4637, f=T30."Disabled and Grayed Out" ("Disabled")) -> (s? t:f=w4636:T30)
                          n2820 = case shown="False" w4635 {
                            tunnel: w4636 -> [w4641 _]
                            tunnel: [w4641 T30."Disabled and Grayed Out" ("Disabled")] -> w4634
                            frame False {
                              # "StationID present"
                            }
                            frame True {
                              # "No StationID"
                            }
                          }
                          n2821 = property on="Report Generate" class="Bool"("DisabledEnum"=w4636) -> ()  [unwired: 2 in, 2 out]
                          n2822 = disable-structure shown="Disabled" {
                            disable-tunnel: w4634 -> [w4640 _]
                            frame Disabled {
                              # "WIll be enabled when user clicks on the FTP List MCListbox"
                              n2823 = property on="cRIO FTP Copy" class="Bool"("DisabledEnum"=w4640) -> ()  [unwired: 2 in, 2 out]
                            }
                            frame Enabled {
                            }
                          }
                          n2824 = property on="cRIO  Search" class="Bool"("DisabledEnum"=w4634) -> ()  [unwired: 2 in, 2 out]
                        }
                      }
                      n2825 = local write "Plant and Furnace Name"(w4622) -> ()
                      n2826 = Concatenate Strings("{Ready to Start}{Update Local Variables From DB}" ("string"), w4512) -> (w4511:string)
                      n2827 = call "Queue - EnQueue to MessageQ.vi"("<NoD> Don't Display to UI"=TRUE, "Message"=w4511) -> ()  [unwired: 9 in, 1 out]
                      n2828 = Unbundle By Name(w4510) -> ("LanguageID"=w4579:string, "PlantID"=w4573:string)
                      n2829 = Concatenate Strings("[UserID] = " ("string"), w4619, ", [UserName] =  " ("string"), w4616, ", [PlantId] =  " ("string"), w4573, ", [SystemId] =  " ("string"), w4529) -> (w4615:string)
                      n2830 = Concatenate Strings("<APP><I 110> " ("string"), w4615) -> (w4614:string)
                      n2831 = call "Queue - EnQueue to MessageQ.vi"("<NoD> Don't Display to UI"=TRUE, "Message"=w4614) -> ()  [unwired: 9 in, 1 out]
                      n2832 = call "DB - [Config].[UnitOfMeasurement].vi"("[UnitOfMeasurementId]"=w4578, "[LanguageId]"=w4579, "[PlantId]"=w4573) -> ("Unit Of Measurement"=w4580:string)  [unwired: 5 in, 3 out]
                      n2833 = local read "Temperature Units"() -> (w4581:refnum<vi>[])
                      n2834 = global write "Global SRTRS.vi" "Temperature Units"(w4580) -> ()
                      n2835 = for {
                        tunnel: w4581 -> [w4647] mode=indexing
                        tunnel: w4580 -> [w4646]
                        n2836 = property class="Str"(reference=w4647, "Value"=w4646) -> (error out=w4645:errorcluster)  [unwired: 1 in, 1 out]
                        n2837 = local write "Property Node Error"(w4645) -> ()
                      }
                      n2838 = Search and Replace String(input string="ni.var.psp://cRIO IP/RT Library" ("String"), search string="cRIO IP" ("String"), replace string=w4556) -> (result string=w4558:string)  [unwired: 5 in, 3 out]
                      n2839 = Search and Replace String(input string="visa://cRIO IP/ASRL1::INSTR" ("String"), search string="cRIO IP" ("String"), replace string=w4556) -> (result string=w4552:string)  [unwired: 5 in, 3 out]
                      n2840 = local read "Use Host COM Port"() -> (w4554:bool)
                      n2841 = local read "Host COM Port"() -> (w4553:string)
                      n2842 = local write "cRIO shared variable RT Library"(w4558) -> ()
                      n2843 = local write "cRIO COM Port"(w4552) -> ()
                      n2844 = local write "cRIO IP"(w4556) -> ()
                      n2845 = Select(t=w4553, s=w4554, f=w4552) -> (s? t:f=w4555:string)
                      n2846 = local write "VISA resource name RS232"(w4555) -> ()
                    }
                    frame 1 {
                      w4650 = T75[] [] items=["GenericSystemId", "ScreenLockTimer", "TimeSyncSchedule", "TimeSyncTolerance", "TransactStartNo"]
                      w4655 = T72[] [] items=["AllowWpsEdit", "ChartSeparation", "DataLogInterval", "DateFormat", "EnableCmsUpdate", "PermittedTempDiff", "PermittedTimeDiff", "StartStopMarker", "DisplayRefChart", "EnableAmsUpdate"]
                      w4700 = 1  # [Value]
                      w4701 = 0  # [SettingId]
                      w4649 = T75[] [enum."GenericSystemId", enum."ScreenLockTimer", enum."TimeSyncSchedule", enum."TimeSyncTolerance", enum."TransactStartNo"] items=["GenericSystemId", "ScreenLockTimer", "TimeSyncSchedule", "TimeSyncTolerance", "TransactStartNo"]
                      w4654 = T72[] [enum."AllowWpsEdit", enum."ChartSeparation", enum."DataLogInterval", enum."DateFormat", enum."EnableCmsUpdate", enum."PermittedTempDiff", enum."PermittedTimeDiff", enum."AllowWpsEdit", enum."StartStopMarker", enum."DisplayRefChart", enum."EnableAmsUpdate"] items=["AllowWpsEdit", "ChartSeparation", "DataLogInterval", "DateFormat", "EnableCmsUpdate", "PermittedTempDiff", "PermittedTimeDiff", "StartStopMarker", "DisplayRefChart", "EnableAmsUpdate"]
                      w4706 = 1  # [Value]
                      w4707 = 0  # [ParameterId]
                      # "No Updates if Empty"
                      # "No Updates if Empty"
                      # "Write Raw Strings?"
                      # "Not Written\ncRIO Folder = \"/c/ni-rt/LabVIEW Data/SRTRS4070\"\ncRIO Data Retention = \"3\"\nFurnace Number = \"03\"\nRunning Number = \"828\"\nHost COM Port = \"COM3\""
                      # "ENUM gives us Actual Name\nGood for Case Structures"
                      # "Write to ini file"
                      n2847 = local read "Show Debug TAB"() -> (w4664:bool)
                      n2848 = property on="Tab Body" class="TabCtl (strict)"() -> ("Pages"=w4666:refnum<vi>[])  [unwired: 2 in, 2 out]
                      n2849 = local read "Lite Version"() -> (w4665:bool)
                      n2850 = for {
                        tunnel: w4666 -> [w4719] mode=indexing
                        tunnel: w4664 -> [w4718]
                        tunnel: w4665 -> [w4715]
                        tunnel: [w4713] -> w4667
                        n2851 = property class="Page"(reference=w4719) -> (reference out=w4714:refnum<vi>, "PageLabel"=w4717:string)  [unwired: 1 in, 1 out]
                        n2852 = case shown="\"Debug\"" w4717 {
                          tunnel: w4718 -> [_ w4722 _ _]
                          tunnel: [w4720 w4722 FALSE TRUE] -> w4716
                          tunnel: w4715 -> [w4721 _ _ _]
                          frame "Execute", "Setup", Default {
                            # "If Lite Version\nthese TAB will be hidden"
                            n2853 = Not(x=w4721) -> (.not. x?=w4720:bool)
                          }
                          frame "Debug" {
                            # "Debug dependent of \n\"Show Report Tab ONLY\""
                          }
                          frame "Logon" {
                          }
                          frame "Master Data", "Report" {
                            # "These Tabs ALWAYS shown"
                          }
                        }
                        n2854 = property class="Page"(reference=w4714, "PageVis"=w4716) -> (error out=w4713:errorcluster)  [unwired: 1 in, 1 out]
                      }
                      n2855 = for {
                        tunnel: w4649 -> [w4793] mode=indexing
                        tunnel: [w4792] -> w4697 mode=indexing
                        n2856 = Format Into String(w4793) -> (resulting string=w4792:string)  [unwired: 3 in, 1 out]
                      }
                      n2857 = global read "Global SRTRS.vi" "Logon"() -> (w4670:T21)
                      n2858 = for {
                        tunnel: w4654 -> [w4795] mode=indexing
                        tunnel: [w4794] -> w4703 mode=indexing
                        n2859 = Format Into String(w4795) -> (resulting string=w4794:string)  [unwired: 3 in, 1 out]
                      }
                      n2860 = Unbundle By Name(w4670) -> ("PlantID"=w4669:string)
                      n2861 = call "DB - [Config].[Parameter].vi"("Application"="SRTRS", "[PlantId]"=w4669, "[ParameterId] Values"=w4703) -> ("2D data"=w4657:string[][])  [unwired: 6 in, 2 out]
                      "[Config].[Parameter]" <- w4657
                      n2862 = call "DB - [Config].[GeneralSetting].vi"("Application"="SRTRS", "[SettingId] Values"=w4697) -> ("2D data"=w4652:string[][])  [unwired: 7 in, 2 out]
                      "[Config].[GeneralSetting]" <- w4652
                      n2863 = Empty Array?(array=w4657) -> (empty?=w4656:bool)
                      n2864 = Index Array(array=w4652, index (col) #1=w4701, index (col) #2=w4700) -> (element #1=w4698:string[], element #2=w4699:string[])  [unwired: 2 in]
                      n2865 = Empty Array?(array=w4652) -> (empty?=w4651:bool)
                      n2866 = call <vilib>:"Application Directory.vi"() -> ("Application Directory"=w4696:path)
                      n2867 = Index Array(array=w4657, index (col) #1=w4707, index (col) #2=w4706) -> (element #1=w4704:string[], element #2=w4708:string[])  [unwired: 2 in]
                      n2868 = Build Path(base path=w4696, name or relative path="SRTRS.ini" ("ini Name")) -> (appended path=w4693:path)
                      n2869 = Select(t=w4650, s=w4651, f=w4649) -> (s? t:f=w4648:T75[])
                      n2870 = Array Size(array="[TabUserAccess]") -> (size(s)=w4663:i32)
                      n2871 = call <vilib>:"Open Config Data.vi"("create file if necessary (T)"=FALSE, "configuration file path"=w4693) -> ("error out"=w4691:errorcluster, "refnum"=w4692:T59)  [unwired: 7 in, 1 out]
                      n2872 = Select(t=w4655, s=w4656, f=w4654) -> (s? t:f=w4653:T72[])
                      n2873 = case shown="0" w4663 {
                        tunnel: [bool[] [TRUE, TRUE, TRUE, FALSE, FALSE] w4712] -> w4661
                        tunnel: "[TabUserAccess]" -> [_ w4712]
                        frame 0 {
                        }
                        frame 1, Default {
                        }
                      }
                      n2874 = flat-sequence {
                        tunnel: w4667 -> [_]
                        tunnel: w4661 -> [w4725]
                        frame #0 {
                          n2875 = control-ref of="Tab Body"() -> (w4728:refnum<vi>)
                          n2876 = call "Tabs - Page Visibility.vi"("Matching Tab#"=i32[] [0, 1, 2, 3, 11, 12], "PageLabel"=string[] ["Setup", "Execute", "Report", "Master Data", "Admin", "Config"], "[TabUserAccess]"=w4725, "TabControl in"=w4728) -> ()  [unwired: 7 in, 1 out]
                        }
                        frame #1 {
                          n2877 = local write "Tab Body"(Enum_-_Tabs."Setup" ("Tab Body")) -> ()
                        }
                      }
                      n2878 = for {
                        tunnel: w4653 -> [w4805] mode=indexing
                        tunnel: w4704 -> [w4809]
                        tunnel: w4708 -> [w4807]
                        tunnel: [w4804] -> w4709
                        tunnel: [w4797] -> w4690
                        tunnel: w4692 -> [w4801]
                        tunnel: w4691 -> [w4803]
                        # "[Config].[Parameters]"
                        n2879 = Format Into String(w4805) -> (resulting string=w4802:string)  [unwired: 3 in, 1 out]
                        n2880 = Search 1D Array(1D array=w4809, element=w4802) -> (index of element=w4808:i32)  [unwired: 1 in]
                        n2881 = Index Array(array=w4807, index=w4808) -> (element=w4806:string)
                        n2882 = case shown="\"DateFormat\"" w4805 {
                          tunnel: w4806 -> [w4829 w4856 w4858 w4862 w4873 w4875 w4877 w4881 w4887 w4891]
                          tunnel: w4802 -> [_ _ _ _ _ _ _ _ _ _]
                          tunnel: ["Edit WPS in Setup" _ "Host Sampling Interval" "Date Format" _ _ "Permitted Temperature Difference" "Permitted Time Difference" "Display Start Stop Marker" "Display Reference Chart"] -> w4800
                          tunnel: [_ _ w4858 w4862 _ _ w4877 w4881 _ _] -> w4799
                          tunnel: [Key_Enum."Boolean" _ Key_Enum."String" Key_Enum."String" _ _ Key_Enum."String" Key_Enum."String" Key_Enum."Boolean" Key_Enum."Boolean"] -> w4798
                          tunnel: [w4826 _ _ _ _ _ _ _ w4884 w4888] -> w4796
                          frame "AllowWpsEdit" {
                            # "The settings are exact copy of that done during in Initialization Sequence"
                            n2883 = flat-sequence "Edit WPS in Setup" {
                              tunnel: w4826 -> [w4830]
                              frame #0 {
                                # "Set according to FLAG from DB"
                                n2884 = control-ref of="MCListBox FHS Master Data"() -> (w4833:refnum<vi>)
                                n2885 = control-ref of="MCListBox FHS Setup"() -> (w4834:refnum<vi>)
                                n2886 = case shown="True" w4830 {
                                tunnel: w4833 -> [w4840 w4842]
                                tunnel: [w4841 w4844] -> w4835
                                tunnel: w4834 -> [_ w4843]
                                frame False {
                                # "Only Master FHS"
                                n2887 = Build Array(w4840) -> (w4841:refnum<vi>[])
                                }
